vi "Usedlinesfromsettingsfile.vi"(0 "sertting":string) -> (1 "used AO names":string[](array[string]), 2 "used AO lines":tag[](array[tag]), 3 "used DO names":string[](array[string]), 4 "used DO lines":tag[](array[tag]))   [LabVIEW 2015]
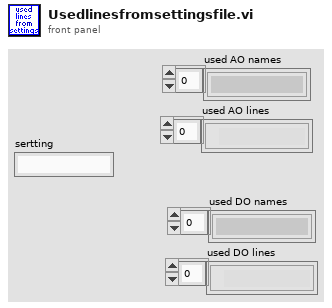
[diagram p1: front panel]
types:
  T1 = cluster{"settings names":string[], "settings locations":path[]}
  T2 = cluster{"used DO lines":tag[], "used DO names":string[]}
  T3 = cluster{"used AO lines":tag[], "used AO names":string[]}
  T4 = typedef "XYZStage.lvlib/XYZStage Configuration.ctl" = cluster{"VISA resource name":refnum<visa-resource-name>, "Timeout (3sec)":u32}
  T5 = cluster{"StageS":i32, "StageL":i32, "currmeas data dir":path, "image OD":u16, "contour OD":u16, "point OD":u16, "AOlines":tag[], "AIlines":tag[], "CI lines":tag[], "DO lines":tag[], "AO names":string[], "CI names":string[], "AI names":string[], "DO names":string[], "CIextensions":string[], "AIextensions":string[], "Voltage to Ygalvo":i32, "Voltage to Xgalvo":i32, "Voltage to patch":i32, "640 shutter":i32, "2P shutter":i32, "LT timestamp":u32, "Vp":i32, "Ip":i32, "camera trigger":i32, "master data dir":path, "voltage to Zpos":i32, "Vto2P":i32, "640 AO":i32, "488 AO":i32, "532 AO":i32, "640TTL":u32, "488TTL":u32, "532TTL":u32, "Device 1 sampleclock out":tag, "Device 1 Starttrigger out":tag, "Device 2 sampleclock in":tag, "Device 2 StartTrigger in ":tag, "2PODTTL":u32, "488 shutter":u32, "LCVR red":u32, "LCVR blue":u32, "Sutter Stage Config":T4}
  T6 = cluster{"newchan":cluster{"String":string, "value":i32}, "ne channel":string}
  T7 = typedef "LVRectTypeDef.ctl" = cluster{"Left":i16, "Top":i16, "Right":i16, "Bottom":i16}
  T8 = cluster{"Xpixels":i32, "Vxminref":dbl, "Vxmaxref":dbl, "P":dbl, "Ypixels":i32, "Vyminref":dbl, "Vymaxref":dbl, "srate":sgl, "sAOxy":i32, "timeout":dbl, "type":string, "date":string, "time":string, "Colormap":u16, "Drawing Mode":u16, "Scanning Mode":u16, "square pixels":bool, "square matrix":bool, "Xpixels Img":i32, "Vx-min Img":dbl, "VX-max Img":dbl, "Ypixels Img":i32, "Vy-min Img":dbl, "Vy-max Img ":dbl, "Angle Img":dbl, "autoshutter":bool, "finite":bool, "cont":bool, "wavdet":bool, "measpoints":i32, "avpp":i32, "bufferAO":i32, "bufferAI":i32, "starttick":u32, "waveform":path, "Vx-ref":dbl, "Vy-ref":dbl, "refreshrate":dbl, "refreshbuffer":i32, "tt_cycles":i32, "motorref":refnum<k7>, "mirrorswitch":refnum<k7>, "sample mode":i32, "maxbufferAI":i32, "srateAODO":sgl, "bin":sgl, "Pel":sgl, "Angle draw":dbl, "srate Img":sgl, "ROIimg_plotbounds":T7, "auto OD":bool, "ODfilt":u16, "aAI":i32[], "aCI":i32[], "aAO":u32[], "aDO":u32[], "refwfsize":dbl, "Lifetime":bool, "Vz-Img":dbl, "Vz-ref":dbl, "Vz-reset":dbl, "AIoverride":bool, "aAS":u32[], "XYZstart":dbl[]}
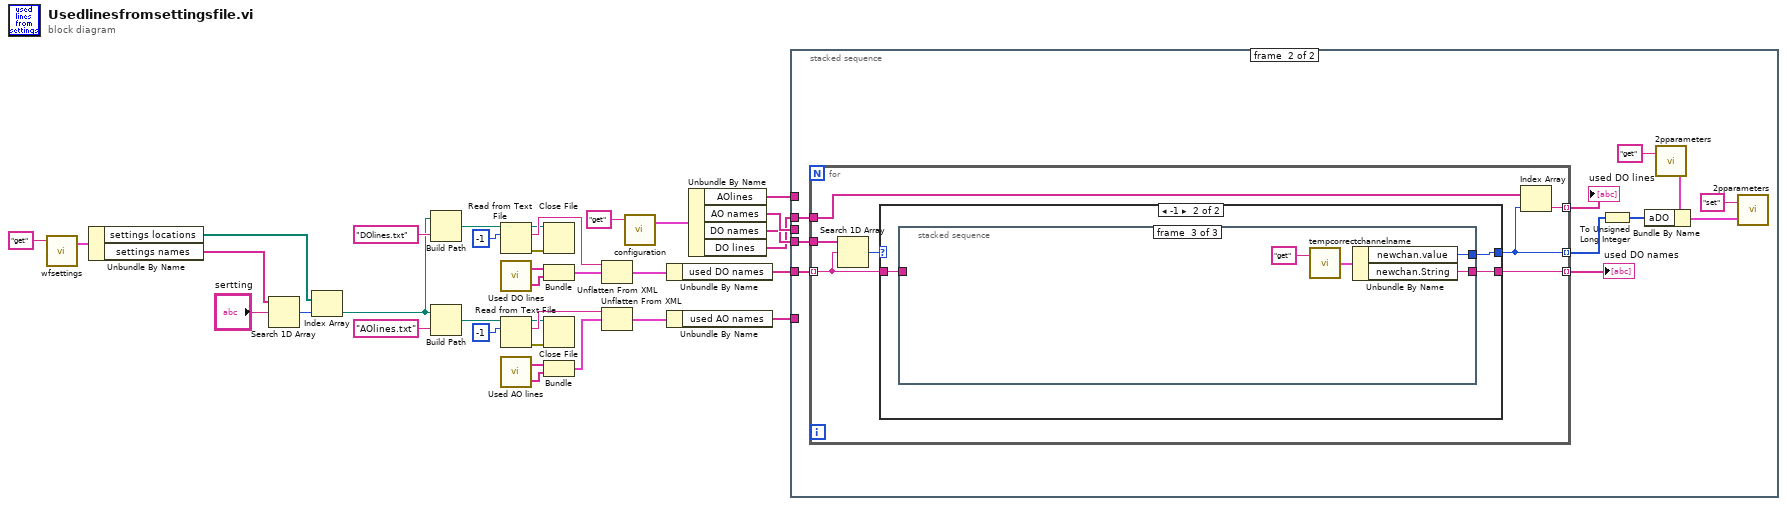
[diagram p0: block diagram]
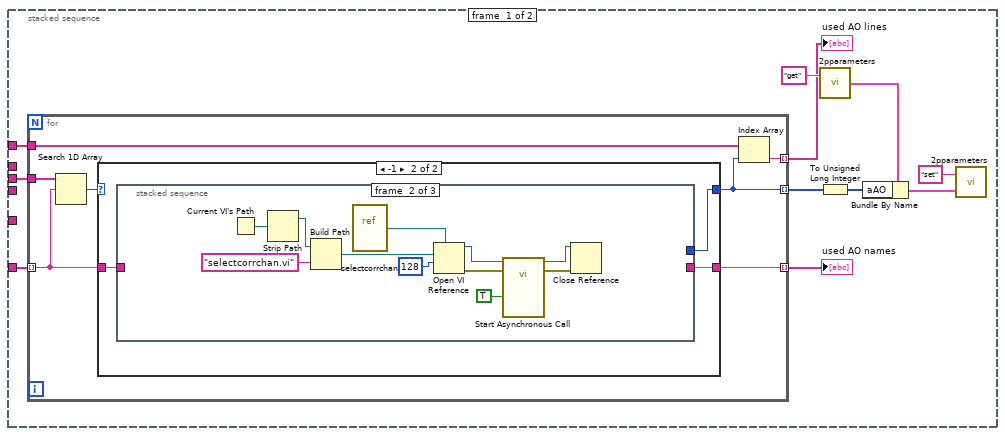
[diagram p2: hidden frame]
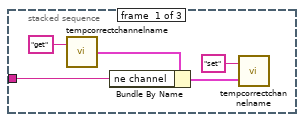
[diagram p4: hidden frame]
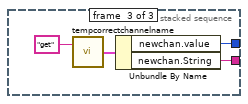
[diagram p5: hidden frame]
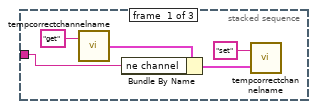
[diagram p7: hidden frame]
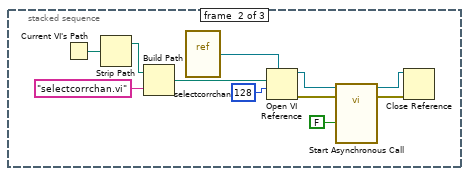
[diagram p8: hidden frame]
diagram:
  n1 = call "wfsettings.vi"("command"="get") -> ("wfsettings out"=w33:T1)  [unwired: 2 in, 1 out]
  n2 = Unbundle By Name(w33) -> ("settings locations"=w31:path[], "settings names"=w32:string[])
  n3 = Search 1D Array(1D array=w32, element="sertting") -> (index of element=w35:i32)  [unwired: 1 in]
  n4 = Index Array(array=w31, index=w35) -> (element=w10:path)
  n5 = Build Path(base path=w10, name or relative path="DOlines.txt") -> (appended path=w12:path)
  n6 = Build Path(base path=w10, name or relative path="AOlines.txt") -> (appended path=w22:path)
  n7 = Read from Text File(file (use dialog)=w12, count=-1) -> (refnum out=w16:refnum<file>, text=w18:string, error out=w17:errorcluster)  [unwired: 2 in, 1 out]
  n8 = call "Used DO lines.vi"() -> ("used DO names"=w19:string[], "used DO lines"=w20:tag[])  [unwired: 2 in]
  n9 = Read from Text File(file (use dialog)=w22, count=-1) -> (refnum out=w27:refnum<file>, text=w29:string, error out=w28:errorcluster)  [unwired: 2 in, 1 out]
  n10 = call "Used AO lines.vi"() -> ("used AO names"=w25:string[], "used AO lines"=w24:tag[])  [unwired: 2 in]
  n11 = Close File(refnum=w16, error in=w17) -> ()  [unwired: 2 out]
  n12 = Bundle("used DO lines"=w20, "used DO names"=w19) -> (w14:T2)  [unwired: 1 in]
  n13 = Close File(refnum=w27, error in=w28) -> ()  [unwired: 2 out]
  n14 = Bundle("used AO lines"=w24, "used AO names"=w25) -> (w30:T3)  [unwired: 1 in]
  n15 = Unflatten From XML(xml string=w18, type=w14) -> (value=w9:T2)  [unwired: 1 in, 1 out]
  n16 = Unflatten From XML(xml string=w29, type=w30) -> (value=w23:T3)  [unwired: 1 in, 1 out]
  n17 = call "configuration.vi"("command"="get") -> ("config out"=w6:T5)  [unwired: 2 in, 1 out]
  n18 = Unbundle By Name(w9) -> ("used DO names"=w3:string[])
  n19 = Unbundle By Name(w23) -> ("used AO names"=w8:string[])
  n20 = Unbundle By Name(w6) -> ("AOlines"=w5:tag[], "AO names"=w4:string[], "DO names"=w2:string[], "DO lines"=w1:tag[])
  n21 = stacked-sequence {
    tunnel: w8 -> [w46 _]
    tunnel: w5 -> [w45 _]
    tunnel: w4 -> [w44 _]
    tunnel: w3 -> [_ w81]
    tunnel: w2 -> [_ w80]
    tunnel: w1 -> [_ w79]
    frame #0 {
      n22 = for {
        tunnel: w46 -> [w51] mode=indexing
        tunnel: w45 -> [w48]
        tunnel: w44 -> [w53]
        tunnel: [w49] -> w39 mode=indexing
        tunnel: [w50] -> w37 mode=indexing
        tunnel: [w47] -> w36 mode=indexing
        n23 = Search 1D Array(1D array=w53, element=w51) -> (index of element=w52:i32)  [unwired: 1 in]
        n24 = case shown="-1" w52 {
          selector: w52 -> [w55 _]
          tunnel: w51 -> [w54 w58]
          tunnel: [w54 w57] -> w50
          tunnel: [w55 w56] -> w49
          frame 0.., Default {
          }
          frame -1 {
            n25 = stacked-sequence {
              tunnel: w58 -> [w60 _ _]
              tunnel: [_ _ w75] -> w57
              tunnel: [_ _ w76] -> w56
              frame #0 {
                n26 = call "tempcorrectchannelname.vi"("command"="get") -> ("param out"=w61:T6)  [unwired: 1 in]
                n27 = Bundle By Name(cluster=w61, "ne channel"=w60) -> (w59:T6)
                n28 = call "tempcorrectchannelname.vi"("param in"=w59, "command"="set") -> ()  [unwired: 1 out]
              }
              frame #1 {
                n29 = Current VI's Path() -> (path=w74:path)
                n30 = Strip Path(path=w74) -> (stripped path=w70:path)  [unwired: 1 out]
                n31 = Build Path(base path=w70, name or relative path="selectcorrchan.vi") -> (appended path=w69:path)
                n32 = vi-ref "selectcorrchan.vi"() -> (w66:refnum<vi>)
                n33 = Open VI Reference(type specifier VI Refnum (for type only)=w66, vi path=w69, options=128) -> (vi reference=w67:refnum<vi>, error out=w72:errorcluster)  [unwired: 3 in]
                n34 = call-by-ref "Start Asynchronous Call"(reference=w67, error in=w72, "AO"=TRUE) -> (reference out=w68:refnum<vi>, error out=w71:errorcluster)
                n35 = Close Reference(reference=w68, error in (no error)=w71) -> ()  [unwired: 1 out]
              }
              frame #2 {
                n36 = call "tempcorrectchannelname.vi"("command"="get") -> ("param out"=w77:T6)  [unwired: 1 in]
                n37 = Unbundle By Name(w77) -> ("newchan.value"=w76:i32, "newchan.String"=w75:string)
              }
            }
          }
        }
        n38 = Index Array(array=w48, index=w49) -> (element=w47:tag)
      }
      "used AO names" <- w37
      "used AO lines" <- w36
      n39 = call "2pparameters.vi"("command"="get") -> ("params out"=w40:T8)  [unwired: 1 in]
      n40 = To Unsigned Long Integer(number=w39) -> (unsigned 32bit integer=w38:u32[])
      n41 = Bundle By Name(cluster=w40, "aAO"=w38) -> (w41:T8)
      n42 = call "2pparameters.vi"("Params in"=w41, "command"="set") -> ()  [unwired: 1 out]
    }
    frame #1 {
      n43 = for {
        tunnel: w81 -> [w94] mode=indexing
        tunnel: w79 -> [w91]
        tunnel: w80 -> [w96]
        tunnel: [w92] -> w85 mode=indexing
        tunnel: [w93] -> w83 mode=indexing
        tunnel: [w90] -> w82 mode=indexing
        n44 = Search 1D Array(1D array=w96, element=w94) -> (index of element=w95:i32)  [unwired: 1 in]
        n45 = case shown="-1" w95 {
          selector: w95 -> [w98 _]
          tunnel: w94 -> [w97 w101]
          tunnel: [w97 w100] -> w93
          tunnel: [w98 w99] -> w92
          frame 0.., Default {
          }
          frame -1 {
            n46 = stacked-sequence {
              tunnel: w101 -> [w103 _ _]
              tunnel: [_ _ w118] -> w100
              tunnel: [_ _ w119] -> w99
              frame #0 {
                n47 = call "tempcorrectchannelname.vi"("command"="get") -> ("param out"=w104:T6)  [unwired: 1 in]
                n48 = Bundle By Name(cluster=w104, "ne channel"=w103) -> (w102:T6)
                n49 = call "tempcorrectchannelname.vi"("param in"=w102, "command"="set") -> ()  [unwired: 1 out]
              }
              frame #1 {
                n50 = Current VI's Path() -> (path=w117:path)
                n51 = Strip Path(path=w117) -> (stripped path=w113:path)  [unwired: 1 out]
                n52 = Build Path(base path=w113, name or relative path="selectcorrchan.vi") -> (appended path=w112:path)
                n53 = vi-ref "selectcorrchan.vi"() -> (w109:refnum<vi>)
                n54 = Open VI Reference(type specifier VI Refnum (for type only)=w109, vi path=w112, options=128) -> (vi reference=w110:refnum<vi>, error out=w115:errorcluster)  [unwired: 3 in]
                n55 = call-by-ref "Start Asynchronous Call"(reference=w110, error in=w115, "AO"=FALSE) -> (reference out=w111:refnum<vi>, error out=w114:errorcluster)
                n56 = Close Reference(reference=w111, error in (no error)=w114) -> ()  [unwired: 1 out]
              }
              frame #2 {
                n57 = call "tempcorrectchannelname.vi"("command"="get") -> ("param out"=w120:T6)  [unwired: 1 in]
                n58 = Unbundle By Name(w120) -> ("newchan.value"=w119:i32, "newchan.String"=w118:string)
              }
            }
          }
        }
        n59 = Index Array(array=w91, index=w92) -> (element=w90:tag)
      }
      "used DO names" <- w83
      "used DO lines" <- w82
      n60 = To Unsigned Long Integer(number=w85) -> (unsigned 32bit integer=w84:u32[])
      n61 = call "2pparameters.vi"("command"="get") -> ("params out"=w86:T8)  [unwired: 1 in]
      n62 = Bundle By Name(cluster=w86, "aDO"=w84) -> (w87:T8)
      n63 = call "2pparameters.vi"("Params in"=w87, "command"="set") -> ()  [unwired: 1 out]
    }
  }
